vi "FL_DEC_split_and_filter_for_saving.vi"(2 "Offset":sgl, 3 "Filter type":u16(ring)=5 items=["None", "Kalman 0.50", "Kalman 0.30", "Kalman 0.12", "Savitzky-Golay 3/5", "Savitzky-Golay 3/11", "Savitzky-Golay 3/31"], 4 "DEC input cluster":T2) -> (1 "Magnets coords":T1)   [LabVIEW 2016]
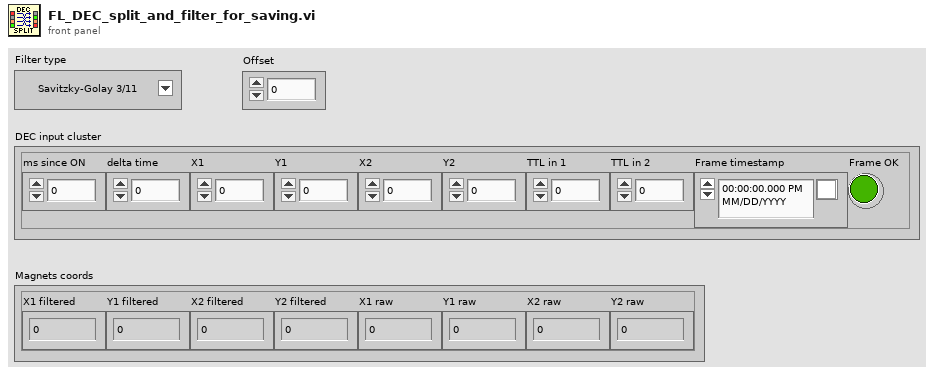
[diagram p1: front panel]
types:
  T1 = cluster{"X1 filtered":dbl, "Y1 filtered":dbl, "X2 filtered":dbl, "Y2 filtered":dbl, "X1 raw":dbl, "Y1 raw":dbl, "X2 raw":dbl, "Y2 raw":dbl}
  T2 = cluster{"ms since ON":u32, "delta time":u32, "X1":sgl, "Y1":sgl, "X2":sgl, "Y2":sgl, "TTL in 1":i16, "TTL in 2":i16, "Frame timestamp":timestamp, "Frame OK":bool}
  T3 = cluster{"X1":dbl, "Y1":dbl, "X2":dbl, "Y2":dbl, "X1":sgl, sgl, "X2":sgl, sgl}
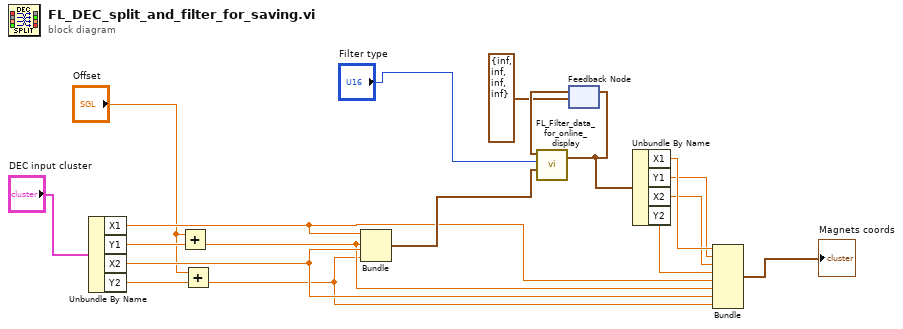
[diagram p0: block diagram]
diagram:
  n1 = Unbundle By Name("DEC input cluster") -> ("X1"=w5:sgl, "Y1"=w8:sgl, "X2"=w4:sgl, "Y2"=w7:sgl)
  n2 = Add(x="Offset", y=w8) -> (x+y=w3:sgl)
  n3 = Add(x="Offset", y=w7) -> (x+y=w2:sgl)
  n4 = Bundle("X1"=w5, w3, "X2"=w4, w2) -> (w15:cluster{"X1":sgl, sgl, "X2":sgl, sgl})  [unwired: 1 in]
  n5 = feedback #1(cluster{"X1":dbl, "Y1":dbl, "X2":dbl, "Y2":dbl} {"X1"=inf, "Y1"=inf, "X2"=inf, "Y2"=inf} ("Output data")) -> (w18:cluster{"X1":dbl, "Y1":dbl, "X2":dbl, "Y2":dbl})
  n6 = call "FL_Filter_data_for_online_display.vi"("Input data"=w15, "Filter type"="Filter type", "Data filtered on previous step"=w18) -> ("Output data"=w14:cluster{"X1":dbl, "Y1":dbl, "X2":dbl, "Y2":dbl})  [unwired: 2 in]
  n7 = feedback-in #1(w14) -> ()
  n8 = Unbundle By Name(w14) -> ("X1"=w12:dbl, "Y1"=w11:dbl, "X2"=w10:dbl, "Y2"=w9:dbl)
  n9 = Bundle("X1"=w12, "Y1"=w11, "X2"=w10, "Y2"=w9, "X1"=w5, w3, "X2"=w4, w2) -> (→"Magnets coords":T3)  [unwired: 1 in]
